vi "Glyph Get CBox.vi"(8 "error in (no error)":errorcluster, 10 "bbox mode":T1(ring), 11 "glyph ref":i64) -> (0 "error out":errorcluster, 2 "BBox":T2, 3 "glyph ref 2":i64)   [LabVIEW 2023, in "Freetype Drawer.lvlib"]
uses:
  Freetype Drawer.lvlib
  libfreetype.dll
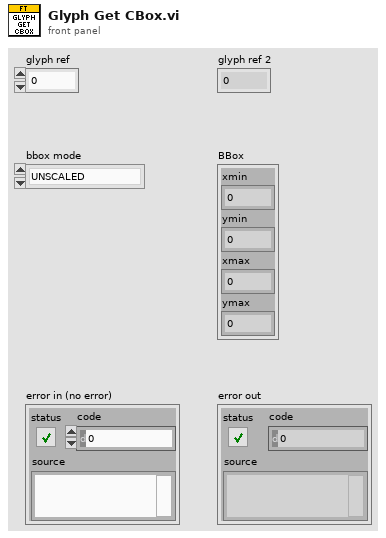
[diagram p1: front panel]
types:
  T1 = enum32{"UNSCALED", "GRIDFIT", "TRUNCATE", "PIXELS"}
  T2 = cluster{"xmin":sgl, "ymin":sgl, "xmax":sgl, "ymax":sgl}
  T3 = cluster{"xmin":i32, "ymin":i32, "xmax":i32, "ymax":i32}
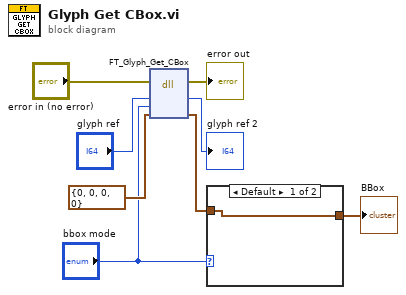
[diagram p0: block diagram]
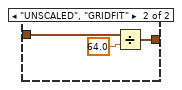
[diagram p2: hidden frame]
diagram:
  n1 = dll-call lib="E:/Labview/LV 2023/Libs/LV Symbol/Freetype Drawer/libfreetype.dll" fn="FT_Glyph_Get_CBox"(error in="error in (no error)", "glyph ref"="glyph ref", "bbox mode"="bbox mode", "acbox"=T3 {"xmin"=0, "ymin"=0, "xmax"=0, "ymax"=0} ("bbox")) -> (error out=→"error out":errorcluster, "glyph ref"=→"glyph ref 2":i64, "acbox"=w7:T3)  [unwired: 4 in, 1 out]
  n2 = case shown="Default" "bbox mode" {
    tunnel: w7 -> [w9 w12]
    tunnel: [w9 w10] -> w3
    frame Default {
    }
    frame "UNSCALED", "GRIDFIT" {
      n3 = Divide(x=w12, y=sgl 64.0) -> (x/y=w10:T2)
    }
  }
  "BBox" <- w3
